vi "Run Service.vi"() -> (0 "error out":errorcluster)   [LabVIEW 2020, in "Game Of Life.lvlib"]
uses:
  Game Of Life.lvlib
  Advanced/Measurement Plugin.lvclass
  <vilib>/Plug-In SDKs/Measurements/NI Measurement Plug-In SDK.lvlib
  C:/Program Files/National Instruments/LabVIEW 2020/vi.lib/Plug-In SDKs/Measurements/Measurement Plugin Service/Measurement Plugin Service.lvclass
  C:/dev/measurementlink-labview/Source/Example Measurements/Game Of Life/Game Of Life/Advanced/Measurement Plugin.lvclass
panel:
  # "Run this VI to start the measurement service.  A window will appear that provides basic information about the running service.\n\nUse the stop button on the window that appears to stop the measurement service."
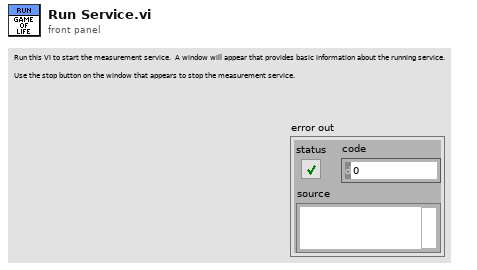
[diagram p1: front panel]
types:
  T1 = enum32{"Invalid", "Standard", "Closed", "Hidden", "Minimized", "Maximized"}
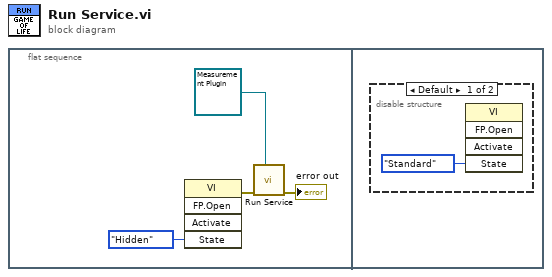
[diagram p0: block diagram]
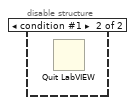
[diagram p2: hidden frame]
diagram:
  n1 = flat-sequence {
    frame #0 {
      n2 = invoke class="VI" method="FP.Open"("State"=T1."Hidden") -> (error out=w3:errorcluster)  [unwired: 4 in, 4 out]
      n3 = call <vilib>:"Run Service.vi"("measurement"=refnum<class "Measurement Plugin.lvclass"> refnum ("MeasurementLink Measurement Template.lvlib:Measurement Customizations.lvclass"), "error in"=w3) -> ("error out"=→"error out":errorcluster)  [unwired: 9 in]
    }
    frame #1 {
      n4 = disable-structure shown="Default" {
        frame condition #0 (active) {
          n5 = invoke class="VI" method="FP.Open"("State"=T1."Standard") -> ()  [unwired: 4 in, 5 out]
        }
        frame condition #1 {
          n6 = Quit LabVIEW() -> ()  [unwired: 1 in]
        }
      }
    }
  }
